vi "max fractional deviation.vi"(9 "max fractional deviation":dbl, 10 "X":dbl, 11 "X'":dbl) -> (3 "In range":bool)   [LabVIEW 2013]
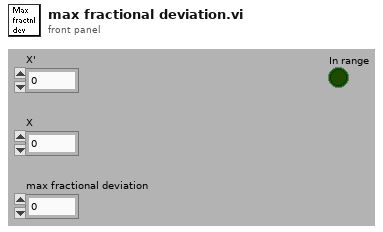
[diagram p1: front panel]
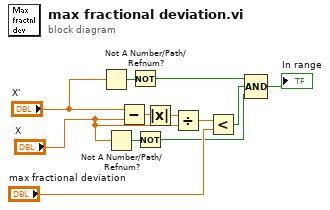
[diagram p0: block diagram]
diagram:
  n1 = Not A Number/Path/Refnum?(number/path/refnum="X'") -> (NaN/Path/Refnum?=w6:bool)
  n2 = Not A Number/Path/Refnum?(number/path/refnum="X") -> (NaN/Path/Refnum?=w7:bool)
  n3 = Subtract(x="X'", y="X") -> (x-y=w8:dbl)
  n4 = Not(x=w6) -> (.not. x?=w4:bool)
  n5 = Not(x=w7) -> (.not. x?=w2:bool)
  n6 = Absolute Value(x=w8) -> (abs(x)=w9:dbl)
  n7 = Divide(x=w9, y="X") -> (x/y=w10:dbl)
  n8 = Less?(x=w10, y="max fractional deviation") -> (x < y?=w3:bool)
  n9 = Compound Arithmetic op=AND(w4, w3, w2) -> (→"In range":bool)
